vi "Update Data.vi"(8 "error in (no error)":errorcluster, 10 "Data Point":dbl, 11 "Report in":refnum<class "Wind TDMS Report.lvclass">) -> (0 "error out":errorcluster, 3 "Report out":refnum<class "Wind TDMS Report.lvclass">)   [LabVIEW 2009, in "Wind TDMS Report.lvclass"]
doc: "This VI is a dynamic dispatch that overrides the parent method.\n\nAAL 9/09"
uses:
  Wind TDMS Report.lvclass
  Wind Report/Wind Report.lvclass
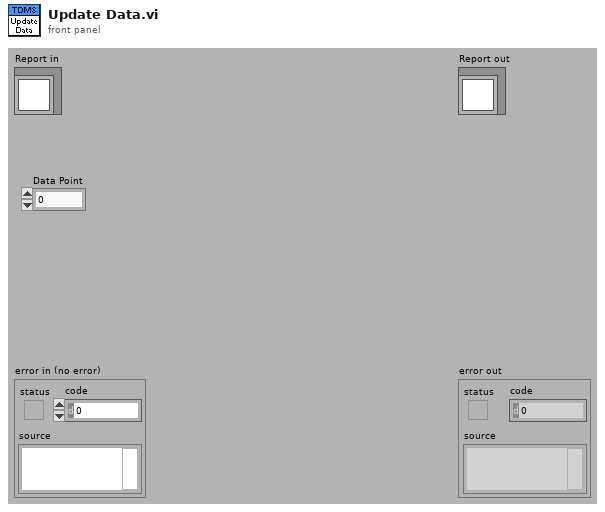
[diagram p1: front panel]
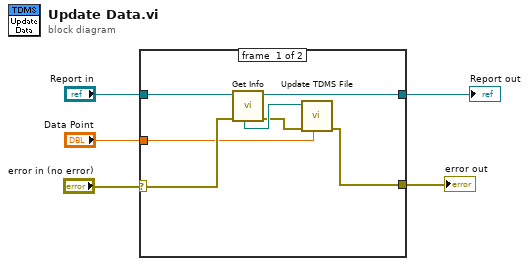
[diagram p0: block diagram]
diagram:
  n1 = case shown="No Error" "error in (no error)" {
    selector: "error in (no error)" -> [w11 w13]
    tunnel: [w7 w13] -> w5
    tunnel: [w6 w14] -> w4
    tunnel: "Report in" -> [w12 w14]
    tunnel: "Data Point" -> [w9 _]
    frame #0 {
      n2 = call "Get Info.vi"("error in (no error)"=w11, "Report.lvclass in"=w12) -> ("error out"=w8:errorcluster, "Report.lvclass out"=w6:refnum<class "Wind TDMS Report.lvclass">, "Path"=w10:path)  [unwired: 3 in, 4 out]
      n3 = call "Update TDMS File.vi"("Data Point"=w9, "error in"=w8, "Path"=w10) -> ("error out"=w7:errorcluster)  [unwired: 8 in]
    }
    frame #1 {
    }
  }
  "error out" <- w5
  "Report out" <- w4
